vi "StoreImage.vi"(0 "reference in":refnum<class "LcPictureBox.lvclass">, 1 "ImageName":string, 2 "ImageNames":string[](array[string]), 3 "ImageFile(Path)":path, 4 "ImageFile(Content)":string, 5 "error in (no error)":errorcluster) -> (14 "reference out":refnum<class "LcPictureBox.lvclass">, 19 "error out":errorcluster)   [LabVIEW 2020, in "LcPictureBox.lvclass"]
uses:
  LcPictureBox.lvclass
  <vilib>/Utility/miscctls.llb/LVMapReplaceAction.ctl
  System.Drawing
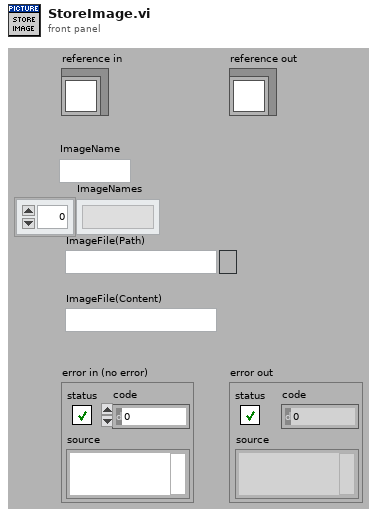
[diagram p1: front panel]
types:
  T1 = typedef "LVMapReplaceAction.ctl" = enum32{"Modify Entry only if found", "Add or Modify Entry", "Delete Entry"}
  T2 = cluster{"ImageOut":refnum<k24>, "ImageSize":cluster{"Width":i32, "Height":i32}}
  T3 = typedef "LcPictureBox.lvclass/ObjectAttributes.ctl" = cluster{"PictureBox":refnum<k24>, "ImageSize":cluster{"Width":i32, "Height":i32}, "PenMemory":map{cluster{"Alpha(100%)":dbl, "Color(Black)":u32, "Pen(Width=1, Solid)":T4}, refnum<k24>}, "GraphicsRef":refnum<k24>, "BrushMemory":map{cluster{"Alpha(100%)":dbl, "Color(Black)":u32}, refnum<k24>}, "Images":refnum<k24>[], "ImageIndex":i32, "BgColor(None)":u32, "LoadedImages":map{string, cluster{"ImageOut":refnum<k24>, "ImageSize":cluster{"Width":i32, "Height":i32}}}, "ColorsMemory":map{cluster{"Alpha(100%)":dbl, "Color(Black)":u32}, refnum<k24>}, "CacheSize":i32, "PictureBoxActiveXReference":refnum<vi>, "Scale":sgl, "Offset":cluster{"x":sgl, "y":sgl}, "zoom_center":cluster{"X":i32, "Y":i32}, "ImagesCreated":refnum<k24>[]}
  T4 = typedef "LcPictureBox.lvclass/Pen.ctl" = cluster{"Width":u16, "Style":enum32{"Solid", "Dash", "Dot", "DashDot", "DashDotDot"}}
  T5 = map{string, cluster{"ImageOut":refnum<k24>, "ImageSize":cluster{"Width":i32, "Height":i32}}}
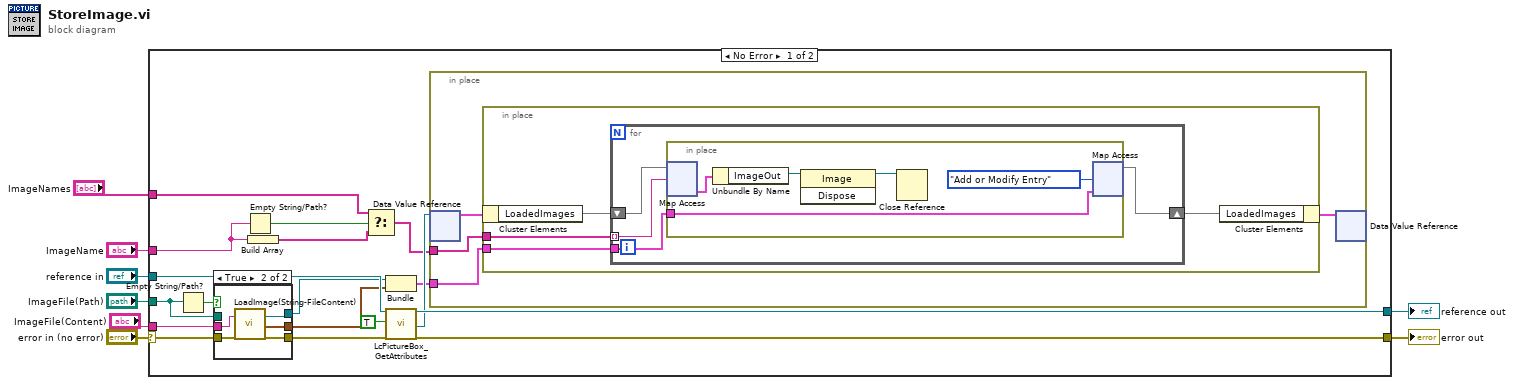
[diagram p0: block diagram]
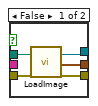
[diagram p2: hidden frame]
diagram:
  n1 = case shown="No Error" "error in (no error)" {
    selector: "error in (no error)" -> [w23 w55]
    tunnel: [w17 w55] -> w7
    tunnel: [w25 w54] -> w5
    tunnel: "reference in" -> [w26 w54]
    tunnel: "ImageFile(Path)" -> [w11 _]
    tunnel: "ImageName" -> [w12 _]
    tunnel: "ImageNames" -> [w15 _]
    tunnel: "ImageFile(Content)" -> [w9 _]
    frame No Error {
      n2 = Empty String/Path?(string/path=w11) -> (empty?=w10:bool)
      n3 = case shown="True" w10 {
        tunnel: w23 -> [w31 w36]
        tunnel: [w30 w35] -> w21
        tunnel: [w29 w34] -> w20
        tunnel: [w28 w33] -> w19
        tunnel: w11 -> [w27 _]
        tunnel: w9 -> [_ w32]
        frame False {
          n4 = call "LoadImage.vi"("ImageFile"=w27, "error in (no error)"=w31) -> ("ImageOut"=w29:refnum<k24>, "ImageSize"=w28:cluster{"Width":i32, "Height":i32}, "error out"=w30:errorcluster)  [unwired: 15 in]
        }
        frame True {
          n5 = call "LoadImage(String-FileContent).vi"("ImageFileContent"=w32, "error in (no error)"=w36) -> ("ImageOut"=w34:refnum<k24>, "ImageSize"=w33:cluster{"Width":i32, "Height":i32}, "error out"=w35:errorcluster)  [unwired: 15 in]
        }
      }
      n6 = Empty String/Path?(string/path=w12) -> (empty?=w16:bool)
      n7 = Build Array(w12) -> (w14:string[])
      n8 = Select(t=w15, s=w16, f=w14) -> (s? t:f=w13:string[])
      n9 = Bundle("ImageOut"=w20, "ImageSize"=w19) -> (w18:T2)  [unwired: 1 in]
      n10 = call "LcPictureBox_GetAttributes.vi"("reference in"=w26, "OnlyGetDvrReference(False)"=TRUE, "error in (no error)"=w21) -> ("reference out"=w25:refnum<class "LcPictureBox.lvclass">, "DataRef"=w22:refnum<data-value>, "error out"=w17:errorcluster)  [unwired: 13 in, 1 out]
      n11 = in-place {
        in-place-border: w18 -> [w38]
        in-place-border: w13 -> [w37]
        n12 = in-place-dvr #1(w22) -> (w40:T3)  [unwired: 1 out]
        n13 = in-place {
          in-place-border: w38 -> [w42]
          in-place-border: w37 -> [w41]
          n14 = in-place-cluster #2(w40) -> ("LoadedImages"=w44:T5)
          n15 = for {
            tunnel: w42 -> [w46]
            tunnel: w41 -> [w45] mode=indexing
            shift-right: [w47] -> w43
            shift-left: w44 -> [w48]
            n16 = in-place {
              in-place-border: w46 -> [w52]
              n17 = in-place-map #3(w48, w45) -> (w51:T2)  [unwired: 1 in, 1 out]
              n18 = Unbundle By Name(w51) -> ("ImageOut"=w50:refnum<k24>)
              n19 = invoke class="Image" method="Dispose"(reference=w50) -> (reference out=w49:refnum<k24>)  [unwired: 2 in, 2 out]
              n20 = Close Reference(reference=w49) -> ()  [unwired: 1 in, 1 out]
              n21 = in-place-map #3(w52, LVMapReplaceAction."Add or Modify Entry" ("action")) -> (w47:T5)  [unwired: 2 out]
            }
          }
          n22 = in-place-cluster #2("LoadedImages"=w43) -> (w39:T3)
        }
        n23 = in-place-dvr #1(w39) -> ()  [unwired: 2 out]
      }
    }
    frame Error {
    }
  }
  "error out" <- w7
  "reference out" <- w5
